vi "数据处理整合 (子VI).vi"(11 "枚举":enum16{"实时数据排序", "小时数据排序"}(ring)) -> (3 "已排序的数组":string[](array[string]))   [LabVIEW 2016, in "数据传输系统.lvlib"]
uses:
  <userlib>/_OpenG.lib/array/array.llb/Remove Duplicates from 1D Array (String)__ogtk.vi
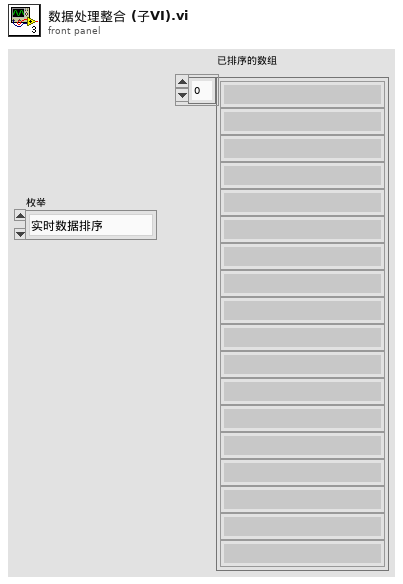
[diagram p1: front panel]
types:
  T1 = cluster{"PH":string[][], "CODCr":string[][], "氨氮":string[][], "CODMn":string[][], "总氮":string[][], "总磷":string[][], "电导率":string[][], "水温":string[][], "DO":string[][], "浊度":string[][], "叶绿素":string[][], "藻密度":string[][], "铜":string[][], "盐度":string[][], "水位":string[][], "流速":string[][], "瞬时流量":string[][], "累积流量":string[][], "亚硝酸盐":string[][], "硫化物":string[][], "ORP":string[][], "铅":string[][], "镉":string[][], "锌":string[][], "镍":string[][], "锰":string[][], "汞":string[][]}
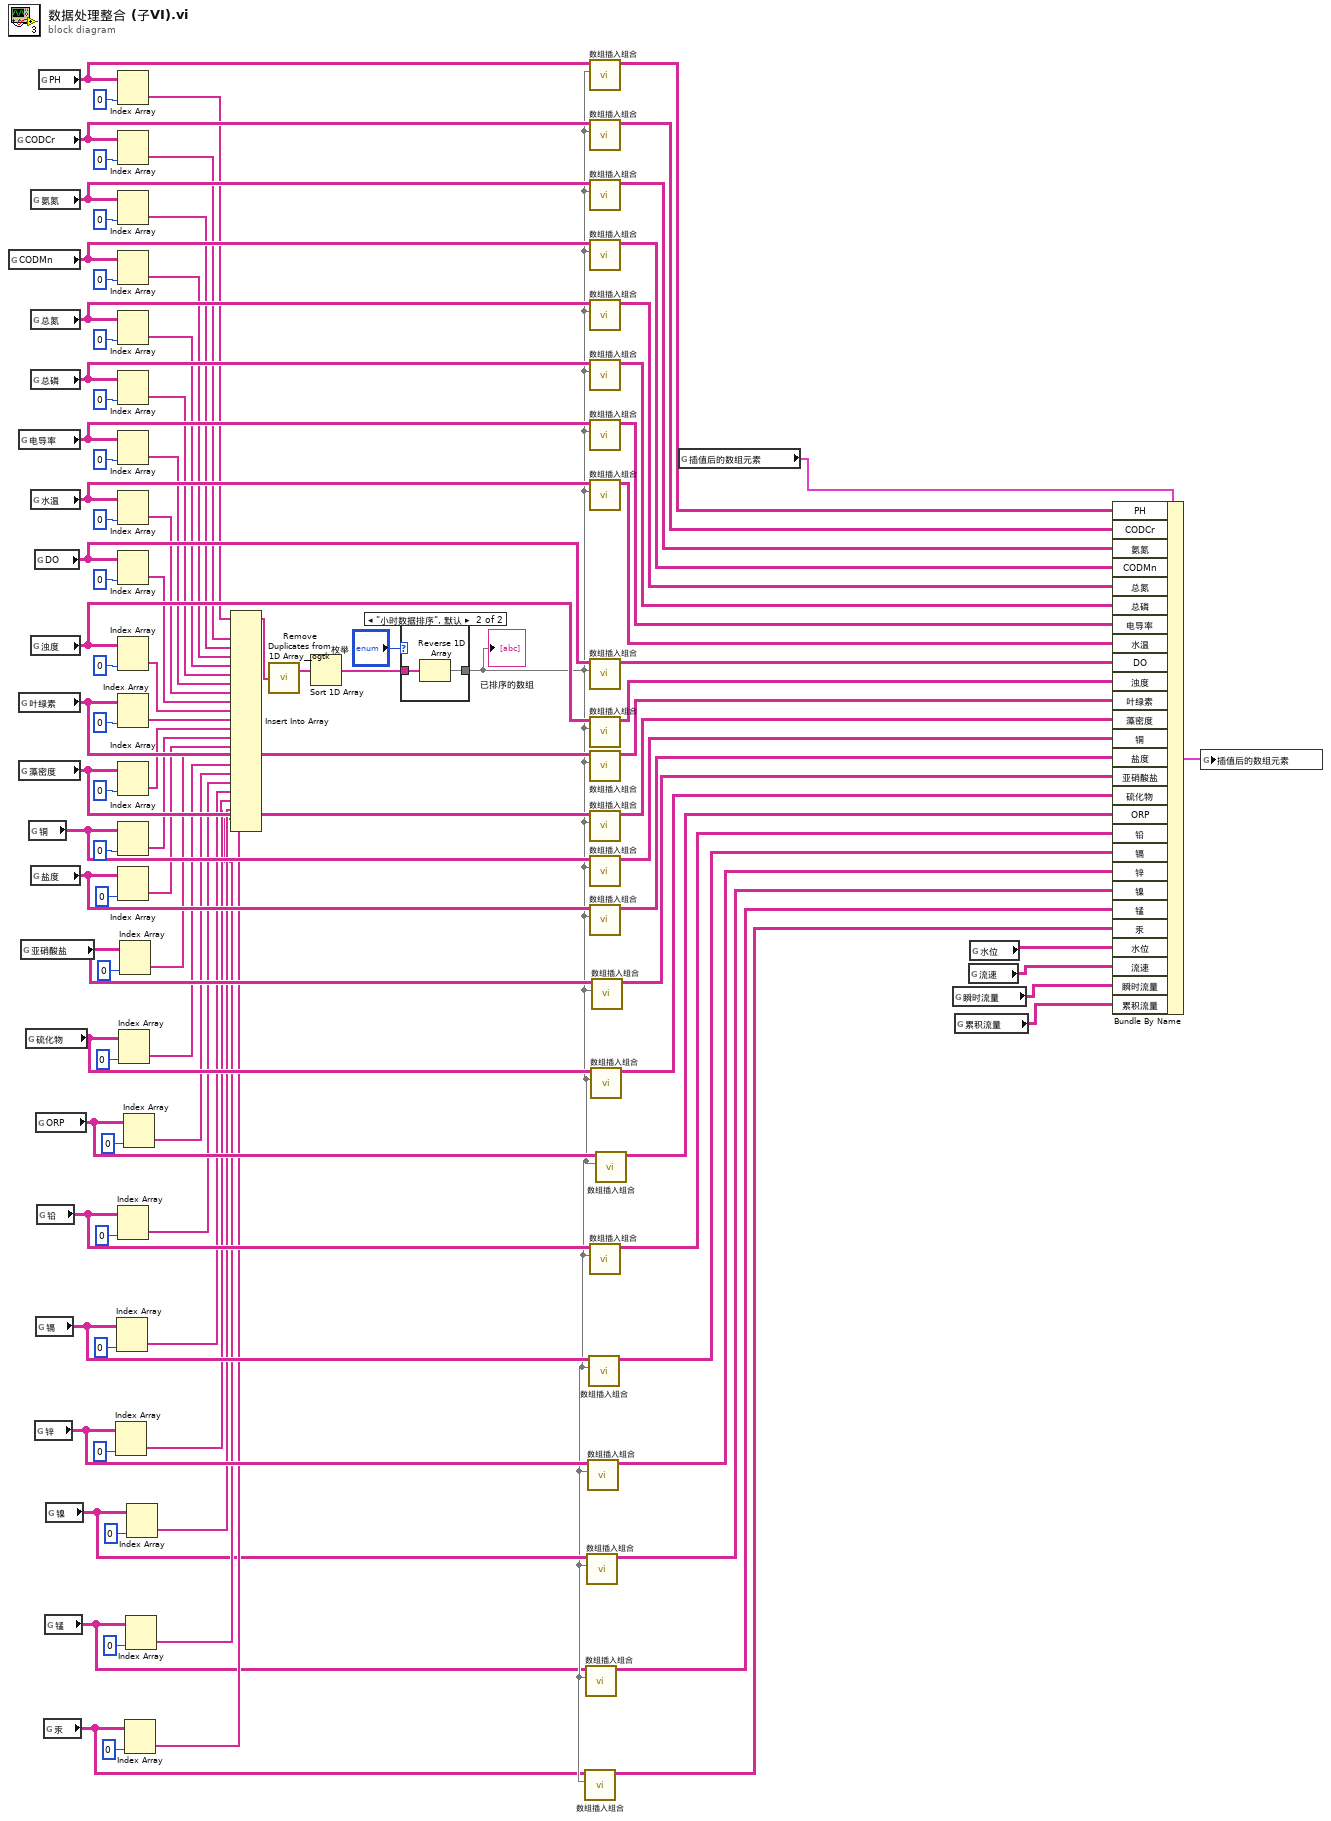
[diagram p0: block diagram]
diagram:
  n1 = global read "全局 所有参数.vi" "CODMn"() -> (w84:string[][])
  n2 = global read "全局 所有参数.vi" "CODCr"() -> (w82:string[][])
  n3 = global read "全局 所有参数.vi" "电导率"() -> (w87:string[][])
  n4 = global read "全局 所有参数.vi" "叶绿素"() -> (w91:string[][])
  n5 = global read "全局 所有参数.vi" "藻密度"() -> (w92:string[][])
  n6 = global read "全局 所有参数.vi" "亚硝酸盐"() -> (w41:string[][])
  n7 = global read "全局 所有参数.vi" "硫化物"() -> (w40:string[][])
  n8 = global read "全局 所有参数.vi" "铜"() -> (w51:string[][])
  n9 = global read "全局 所有参数.vi" "氨氮"() -> (w83:string[][])
  n10 = global read "全局 所有参数.vi" "总氮"() -> (w85:string[][])
  n11 = global read "全局 所有参数.vi" "总磷"() -> (w86:string[][])
  n12 = global read "全局 所有参数.vi" "水温"() -> (w88:string[][])
  n13 = global read "全局 所有参数.vi" "浊度"() -> (w90:string[][])
  n14 = global read "全局 所有参数.vi" "盐度"() -> (w50:string[][])
  n15 = global read "全局 所有参数.vi" "DO"() -> (w89:string[][])
  n16 = global read "全局 所有参数.vi" "锌"() -> (w25:string[][])
  n17 = global read "全局 所有参数.vi" "ORP"() -> (w37:string[][])
  n18 = global read "全局 所有参数.vi" "镉"() -> (w26:string[][])
  n19 = global read "全局 所有参数.vi" "铅"() -> (w29:string[][])
  n20 = global read "全局 所有参数.vi" "PH"() -> (w80:string[][])
  n21 = global read "全局 所有参数.vi" "汞"() -> (w8:string[][])
  n22 = global read "全局 所有参数.vi" "锰"() -> (w9:string[][])
  n23 = global read "全局 所有参数.vi" "镍"() -> (w11:string[][])
  n24 = Index Array(array=w25, index (col)=0 ("索引 (行)")) -> (element=w18:string[])  [unwired: 1 in]
  n25 = Index Array(array=w26, index (col)=0 ("索引 (行)")) -> (element=w19:string[])  [unwired: 1 in]
  n26 = Index Array(array=w80, index (col)=0 ("索引 (行)")) -> (element=w67:string[])  [unwired: 1 in]
  n27 = Index Array(array=w82, index (col)=0 ("索引 (行)")) -> (element=w68:string[])  [unwired: 1 in]
  n28 = Index Array(array=w83, index (col)=0 ("索引 (行)")) -> (element=w69:string[])  [unwired: 1 in]
  n29 = Index Array(array=w84, index (col)=0 ("索引 (行)")) -> (element=w70:string[])  [unwired: 1 in]
  n30 = Index Array(array=w85, index (col)=0 ("索引 (行)")) -> (element=w71:string[])  [unwired: 1 in]
  n31 = Index Array(array=w86, index (col)=0 ("索引 (行)")) -> (element=w72:string[])  [unwired: 1 in]
  n32 = Index Array(array=w87, index (col)=0 ("索引 (行)")) -> (element=w73:string[])  [unwired: 1 in]
  n33 = Index Array(array=w88, index (col)=0 ("索引 (行)")) -> (element=w74:string[])  [unwired: 1 in]
  n34 = Index Array(array=w89, index (col)=0 ("索引 (行)")) -> (element=w75:string[])  [unwired: 1 in]
  n35 = Index Array(array=w90, index (col)=0 ("索引 (行)")) -> (element=w76:string[])  [unwired: 1 in]
  n36 = Index Array(array=w91, index (col)=0 ("索引 (行)")) -> (element=w77:string[])  [unwired: 1 in]
  n37 = Index Array(array=w92, index (col)=0 ("索引 (行)")) -> (element=w78:string[])  [unwired: 1 in]
  n38 = Index Array(array=w51, index (col)=0 ("索引 (行)")) -> (element=w49:string[])  [unwired: 1 in]
  n39 = Index Array(array=w50, index (col)=0 ("索引 (行)")) -> (element=w48:string[])  [unwired: 1 in]
  n40 = Index Array(array=w29, index (col)=0 ("索引 (行)")) -> (element=w20:string[])  [unwired: 1 in]
  n41 = Index Array(array=w40, index (col)=0 ("索引 (行)")) -> (element=w32:string[])  [unwired: 1 in]
  n42 = Index Array(array=w41, index (col)=0 ("索引 (行)")) -> (element=w31:string[])  [unwired: 1 in]
  n43 = Index Array(array=w37, index (col)=0 ("索引 (行)")) -> (element=w33:string[])  [unwired: 1 in]
  n44 = Index Array(array=w8, index (col)=0 ("索引 (行)")) -> (element=w12:string[])  [unwired: 1 in]
  n45 = Index Array(array=w9, index (col)=0 ("索引 (行)")) -> (element=w13:string[])  [unwired: 1 in]
  n46 = Index Array(array=w11, index (col)=0 ("索引 (行)")) -> (element=w14:string[])  [unwired: 1 in]
  n47 = Insert Into Array(array=w67, new element #1=w68, new element #2=w69, new element #3=w70, new element #4=w71, new element #5=w72, new element #6=w73, new element #7=w74, new element #8=w75, new element #9=w76, new element #10=w77, new element #11=w78, new element #12=w49, new element #13=w48, new element #14=w31, new element #15=w32, new element #16=w33, new element #17=w20, new element #18=w19, new element #19=w18, new element #20=w14, new element #21=w13, new element #22=w12) -> (w79:string[])  [unwired: 1 in]
  n48 = call-poly <userlib>:"Remove Duplicates from 1D Array__ogtk.vi"("Input Array"=w79) -> ("Output Array"=w66:string[])  [unwired: 1 out]
  n49 = Sort 1D Array(array=w66) -> (sorted array=w52:string[])
  n50 = case shown="\"小时数据排序\", 默认" "枚举" {
    tunnel: w52 -> [w104 w106]
    tunnel: [w104 w105] -> w10
    frame "实时数据排序" {
    }
    frame "小时数据排序", Default {
      n51 = Reverse 1D Array(array=w106) -> (reversed array=w105:string[])
    }
  }
  "已排序的数组" <- w10
  n52 = call "数组插入组合.vi"("排序后的一维数组"=w10, "输入数组"=w8) -> ("输出结果"=w5:string[][])  [unwired: 9 in]
  n53 = call "数组插入组合.vi"("排序后的一维数组"=w10, "输入数组"=w9) -> ("输出结果"=w6:string[][])  [unwired: 9 in]
  n54 = call "数组插入组合.vi"("排序后的一维数组"=w10, "输入数组"=w11) -> ("输出结果"=w7:string[][])  [unwired: 9 in]
  n55 = call "数组插入组合.vi"("排序后的一维数组"=w10, "输入数组"=w25) -> ("输出结果"=w21:string[][])  [unwired: 9 in]
  n56 = call "数组插入组合.vi"("排序后的一维数组"=w10, "输入数组"=w26) -> ("输出结果"=w22:string[][])  [unwired: 9 in]
  n57 = call "数组插入组合.vi"("排序后的一维数组"=w10, "输入数组"=w80) -> ("输出结果"=w81:string[][])  [unwired: 9 in]
  n58 = call "数组插入组合.vi"("排序后的一维数组"=w10, "输入数组"=w82) -> ("输出结果"=w93:string[][])  [unwired: 9 in]
  n59 = call "数组插入组合.vi"("排序后的一维数组"=w10, "输入数组"=w83) -> ("输出结果"=w94:string[][])  [unwired: 9 in]
  n60 = call "数组插入组合.vi"("排序后的一维数组"=w10, "输入数组"=w84) -> ("输出结果"=w95:string[][])  [unwired: 9 in]
  n61 = call "数组插入组合.vi"("排序后的一维数组"=w10, "输入数组"=w85) -> ("输出结果"=w96:string[][])  [unwired: 9 in]
  n62 = call "数组插入组合.vi"("排序后的一维数组"=w10, "输入数组"=w86) -> ("输出结果"=w97:string[][])  [unwired: 9 in]
  n63 = call "数组插入组合.vi"("排序后的一维数组"=w10, "输入数组"=w87) -> ("输出结果"=w98:string[][])  [unwired: 9 in]
  n64 = call "数组插入组合.vi"("排序后的一维数组"=w10, "输入数组"=w88) -> ("输出结果"=w99:string[][])  [unwired: 9 in]
  n65 = call "数组插入组合.vi"("排序后的一维数组"=w10, "输入数组"=w89) -> ("输出结果"=w100:string[][])  [unwired: 9 in]
  n66 = call "数组插入组合.vi"("排序后的一维数组"=w10, "输入数组"=w90) -> ("输出结果"=w101:string[][])  [unwired: 9 in]
  n67 = call "数组插入组合.vi"("排序后的一维数组"=w10, "输入数组"=w91) -> ("输出结果"=w102:string[][])  [unwired: 9 in]
  n68 = call "数组插入组合.vi"("排序后的一维数组"=w10, "输入数组"=w92) -> ("输出结果"=w103:string[][])  [unwired: 9 in]
  n69 = call "数组插入组合.vi"("排序后的一维数组"=w10, "输入数组"=w51) -> ("输出结果"=w47:string[][])  [unwired: 9 in]
  n70 = call "数组插入组合.vi"("排序后的一维数组"=w10, "输入数组"=w50) -> ("输出结果"=w46:string[][])  [unwired: 9 in]
  n71 = call "数组插入组合.vi"("排序后的一维数组"=w10, "输入数组"=w29) -> ("输出结果"=w23:string[][])  [unwired: 9 in]
  n72 = call "数组插入组合.vi"("排序后的一维数组"=w10, "输入数组"=w40) -> ("输出结果"=w34:string[][])  [unwired: 9 in]
  n73 = call "数组插入组合.vi"("排序后的一维数组"=w10, "输入数组"=w41) -> ("输出结果"=w36:string[][])  [unwired: 9 in]
  n74 = call "数组插入组合.vi"("排序后的一维数组"=w10, "输入数组"=w37) -> ("输出结果"=w35:string[][])  [unwired: 9 in]
  n75 = global read "插值后的新数组.vi" "插值后的数组元素"() -> (w43:T1)
  n76 = global read "全局 所有参数.vi" "瞬时流量"() -> (w2:string[][])
  n77 = global read "全局 所有参数.vi" "累积流量"() -> (w1:string[][])
  n78 = global read "全局 所有参数.vi" "流速"() -> (w3:string[][])
  n79 = global read "全局 所有参数.vi" "水位"() -> (w4:string[][])
  n80 = Bundle By Name(cluster=w43, "PH"=w81, "CODCr"=w93, "氨氮"=w94, "CODMn"=w95, "总氮"=w96, "总磷"=w97, "电导率"=w98, "水温"=w99, "DO"=w100, "浊度"=w101, "叶绿素"=w102, "藻密度"=w103, "铜"=w47, "盐度"=w46, "亚硝酸盐"=w36, "硫化物"=w34, "ORP"=w35, "铅"=w23, "镉"=w22, "锌"=w21, "镍"=w7, "锰"=w6, "汞"=w5, "水位"=w4, "流速"=w3, "瞬时流量"=w2, "累积流量"=w1) -> (w30:T1)
  n81 = global write "插值后的新数组.vi" "插值后的数组元素"(w30) -> ()
